vi "Remove Nan and replace with nearest float.vi"(1 "Unfiltered":dbl[](array[numeric])) -> (0 "Filtered Data":dbl[](array[numeric]))   [LabVIEW 2009]
panel:
  out "Numeric":i32
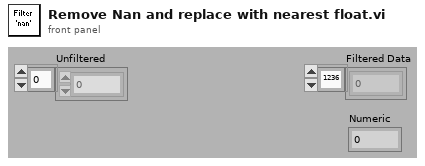
[diagram p1: front panel]
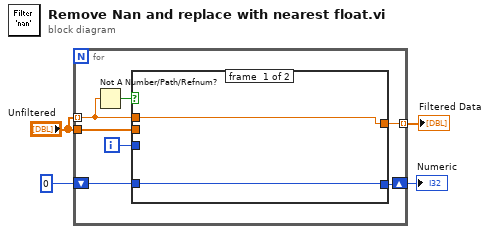
[diagram p0: block diagram]
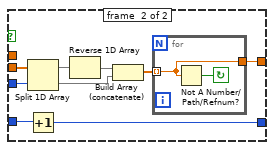
[diagram p2: hidden frame]
diagram:
  n1 = for {
    tunnel: "Unfiltered" -> [w10] mode=indexing
    tunnel: "Unfiltered" -> [w8]
    tunnel: [w9] -> w4 mode=indexing
    shift-right: [w5] -> w1
    shift-left: 0 -> [w6]
    i -> [w7]
    n2 = Not A Number/Path/Refnum?(number/path/refnum=w10) -> (NaN/Path/Refnum?=w11:bool)
    n3 = case shown="True" w11 {
      tunnel: w10 -> [w13 _]
      tunnel: [w13 w20] -> w9
      tunnel: w8 -> [_ w22]
      tunnel: w7 -> [_ w19]
      tunnel: w6 -> [w12 w18]
      tunnel: [w12 w17] -> w5
      frame #0 {
      }
      frame #1 {
        n4 = Split 1D Array(array=w22, index=w19) -> (first subarray=w21:dbl[], second subarray=w15:dbl[])
        n5 = Increment(x=w18) -> (x+1=w17:i32)
        n6 = Reverse 1D Array(array=w21) -> (reversed array=w16:dbl[])
        n7 = Build Array (concatenate)(w16, w15) -> (w14:dbl[])
        n8 = for {
          tunnel: w14 -> [w24] mode=indexing
          tunnel: [w24] -> w20
          stop <- w23 continue-if-true
          n9 = Not A Number/Path/Refnum?(number/path/refnum=w24) -> (NaN/Path/Refnum?=w23:bool)
        }
      }
    }
  }
  "Filtered Data" <- w4
  "Numeric" <- w1
